vi "ActOnEnable.vi"(0 "ActionBase in":refnum<class "ActionBase.lvclass">, 1 "Data":variant, 5 "error in (no error)":errorcluster) -> (14 "ActionBase out":refnum<class "ActionBase.lvclass">, 19 "error out":errorcluster)   [LabVIEW 2017, in "ActionBase.lvclass"]
doc: "Base class implementation (empty)."
uses:
  ActionBase.lvclass
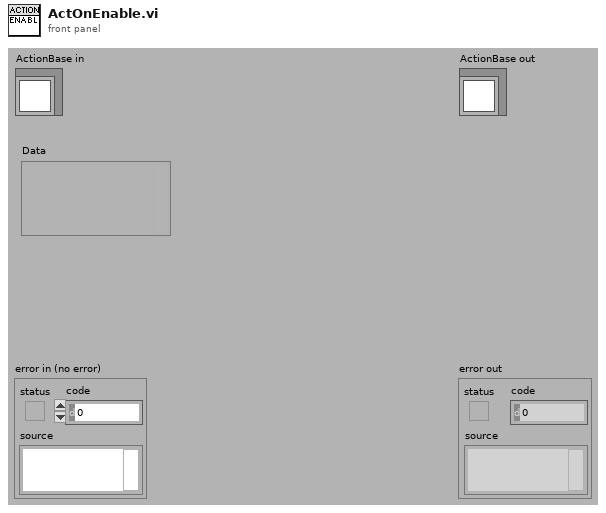
[diagram p1: front panel]
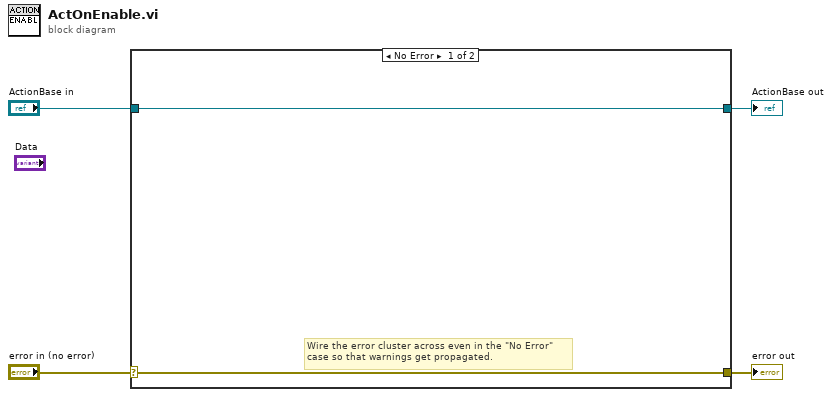
[diagram p0: block diagram]
diagram:
  n1 = case shown="No Error" "error in (no error)" {
    selector: "error in (no error)" -> [w5 w8]
    tunnel: [w5 w8] -> w3
    tunnel: [w6 w7] -> w1
    tunnel: "ActionBase in" -> [w6 w7]
    frame No Error {
      # "Wire the error cluster across even in the \"No Error\"\ncase so that warnings get propagated."
    }
    frame Error {
    }
  }
  "error out" <- w3
  "ActionBase out" <- w1
